vi "截取图像二值化自动调阈值.vi"(1 "白点百分比（0-100）默认50":dbl, 2 "Image Dst":T1, 3 "输入image数组（截取灰度）":dbl[][](array[numeric])) -> (0 "Image Out":T1)   [LabVIEW 2017]
uses:
  <vilib>/vision/Image Controls.llb/IMAQ Image.ctl
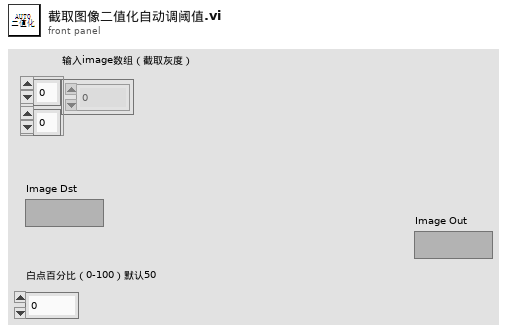
[diagram p1: front panel]
types:
  T1 = typedef "IMAQ Image.ctl" = refnum<image>
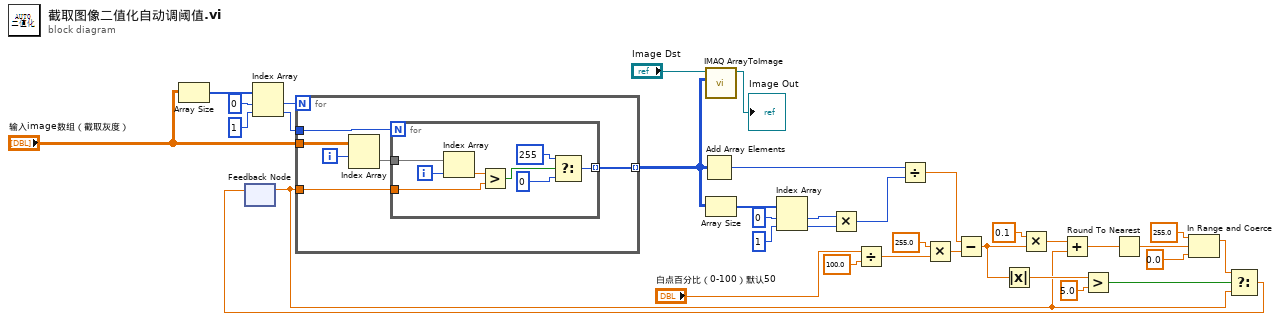
[diagram p0: block diagram]
diagram:
  n1 = Array Size(array="输入image数组（截取灰度）") -> (size(s)=w33:i32[])
  n2 = feedback #1() -> (w2:dbl)  [unwired: 1 in]
  n3 = Index Array(array=w33, index #1=0 ("索引"), index #2=1 ("索引")) -> (element #1=w32:i32, element #2=w29:i32)
  n4 = for {
    N: w32 -> [_]
    tunnel: "输入image数组（截取灰度）" -> [w41]
    tunnel: w29 -> [w39]
    tunnel: [w37] -> w1 mode=indexing
    tunnel: w2 -> [w36]
    i -> [w40]
    n5 = Index Array(array=w41, index (row)=w40) -> (element=w38:dbl[])  [unwired: 1 in]
    n6 = for {
      N: w39 -> [_]
      tunnel: w38 -> [w49]
      tunnel: [w45] -> w37 mode=indexing
      tunnel: w36 -> [w42]
      i -> [w48]
      n7 = Index Array(array=w49, index=w48) -> (element=w47:dbl)
      n8 = Greater?(x=w47, y=w42) -> (0:w46:bool)
      n9 = Select(t=255, s=w46, f=0) -> (s? t:f=w45:i32)
    }
  }
  n10 = Add Array Elements(numeric array=w1) -> (sum=w23:i32)
  n11 = call "IMAQ ArrayToImage"("Image Pixels (U8)"=w1, "Image"="Image Dst") -> ("Image Out"=→"Image Out":T1)  [unwired: 4 in, 5 out]
  n12 = Array Size(array=w1) -> (size(s)=w28:i32[])
  n13 = Index Array(array=w28, index #1=0, index #2=1) -> (element #1=w25:i32, element #2=w24:i32)
  n14 = Multiply(x=w25, y=w24) -> (x*y=w22:i32)
  n15 = Divide(x="白点百分比（0-100）默认50", y=100.0) -> (x/y=w16:dbl)
  n16 = Divide(x=w23, y=w22) -> (x/y=w7:dbl)
  n17 = Multiply(x=255.0, y=w16) -> (x*y=w6:dbl)
  n18 = Subtract(x=w7, y=w6) -> (x-y=w9:dbl)
  n19 = Absolute Value(x=w9) -> (abs(x)=w8:dbl)
  n20 = Multiply(x=0.1, y=w9) -> (x*y=w12:dbl)
  n21 = Add(x=w12, y=w2) -> (x+y=w11:dbl)
  n22 = Greater?(x=w8, y=5.0) -> (0:w14:bool)
  n23 = Round To Nearest(number=w11) -> (nearest integer value=w19:dbl)
  n24 = In Range and Coerce(upper limit=255.0, x=w19, lower limit=0.0) -> (coerced(x)=w10:dbl)  [unwired: 1 out]
  n25 = Select(t=w10, s=w14, f=w2) -> (s? t:f=w3:dbl)
  n26 = feedback-in #1(w3) -> ()
